vi "Specify Windows LabVIEW Runtime.vi"(8 "error in (no error)":errorcluster, 11 "LabVIEW Runtime Path (.exe,.dll)":path) -> (0 "error out":errorcluster)   [LabVIEW 2020, in "common.lvlib"]
doc: "This VI is only required for situations on Windows where multiple LabVIEW runtimes are in use simultaneously within the same context for example when LabVIEW code is being called in TestStand.\n\nEnsure this VI is called before any other calls to this toolkit to ensure the LabVIEW runtime is correctly set and the correct internal resources are loaded."
uses:
  common.lvlib
  bin/gartoolkit_32-1.dll
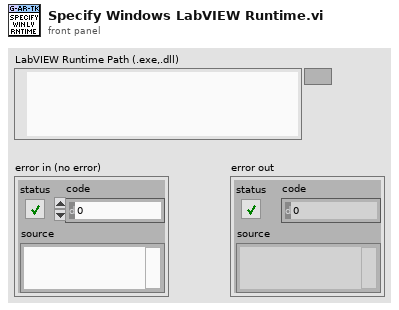
[diagram p1: front panel]
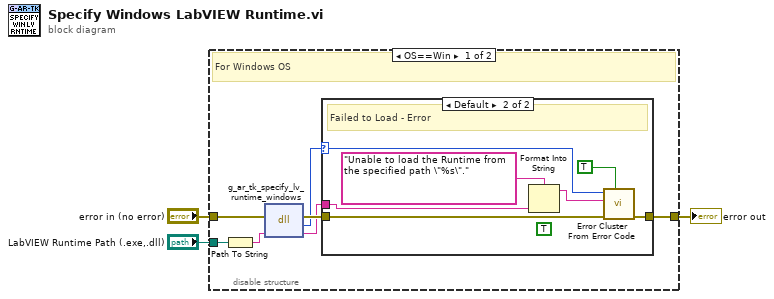
[diagram p0: block diagram]
diagram:
  n1 = disable-structure shown="OS==Win" {
    disable-tunnel: "error in (no error)" -> [w7 w19]
    disable-tunnel: [w6 w19] -> w2
    disable-tunnel: "LabVIEW Runtime Path (.exe,.dll)" -> [w5 _]
    frame condition #0 (active) {
      # "For Windows OS"
      n2 = Path To String(path=w5) -> (string=w10:string)
      n3 = dll-call lib="C:/serenial/lib/g-augmented-reality-toolkit/LabVIEW/common/bin/gartoolkit_*-1.*" fn="g_ar_tk_specify_lv_runtime_windows"(error in=w7, "arg1"=w10) -> (error out=w9:errorcluster, "mg_err_code"=w8:i32, "arg1"=w4:string)  [unwired: 2 in, 1 out]
      n4 = case shown="Default" w8 {
        selector: w8 -> [_ w17]
        tunnel: w9 -> [w11 w18]
        tunnel: [w11 w16] -> w6
        tunnel: w4 -> [_ w14]
        frame 0 {
          # "Loaded OK"
        }
        frame Default {
          (unwired) TRUE ("show call chain? (False)")
          # "Failed to Load - Error"
          n5 = Format Into String(format string="Unable to load the Runtime from the specified path \"%s\".", w14) -> (resulting string=w13:string)  [unwired: 2 in, 1 out]
          n6 = call <vilib>:"Error Cluster From Error Code.vi"("show call chain? (False)"=TRUE, "error in (no error)"=w18, "error message (\"\")"=w13, "error code (0)"=w17) -> ("error out"=w16:errorcluster)  [unwired: 5 in]
        }
      }
    }
    frame condition #1 {
      # "No Call on Non-Win OSs"
    }
  }
  "error out" <- w2
